vi "Pico_PassFail.vi"(11 "Booléen":bool) -> (3 "Vout":string)   [LabVIEW 2020]
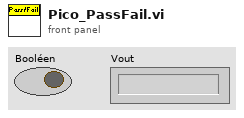
[diagram p1: front panel]
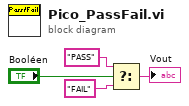
[diagram p0: block diagram]
diagram:
  n1 = Select(t="PASS", s="Booléen", f="FAIL") -> (s? t:f=→"Vout":string)
